vi "XY Graph Cumulative Function of Multiple Plots.vi"(8 "error in (no error)":errorcluster, 10 "Selected Plots":i32[](array[numeric]), 11 "Selected Plot Info":T1) -> (0 "error out":errorcluster, 1 "Cumulative Function Plot Message":string, 3 "Last Cumulative Function Plot":cluster{"t Array":dbl[], "IRF Array":dbl[]}, 4 "Single Plot?":bool)   [LabVIEW 2021, in "XY Graph Add-Ons.lvlib"]
uses:
  XY Graph Add-Ons.lvlib
  XY Graph Selected Plot Info.ctl
  XY Graph Refnum.ctl
  <vilib>/Utility/miscctls.llb/LVPoint32TypeDef.ctl
  Strings/Strings.lvlib
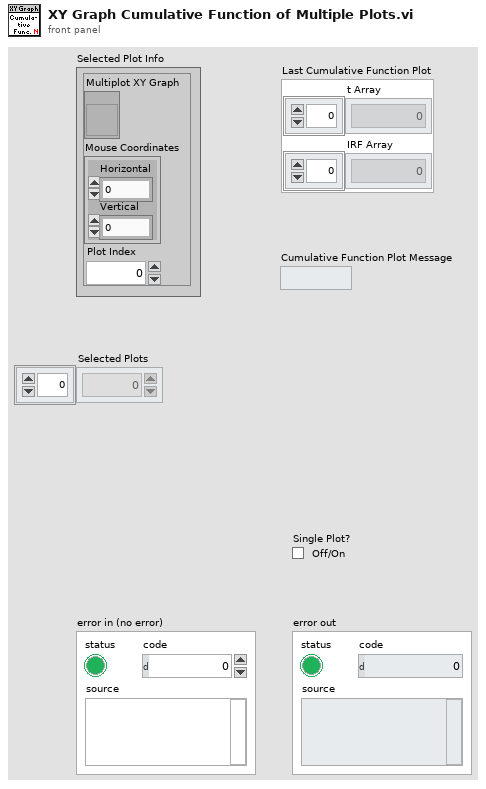
[diagram p1: front panel]
types:
  T1 = typedef "XY Graph Add-Ons.lvlib/XY Graph Selected Plot Info.ctl" = cluster{"Multiplot XY Graph":T2, "Mouse Coordinates":T3, "Plot Index":i32}
  T2 = typedef "XY Graph Add-Ons.lvlib/XY Graph Refnum.ctl" = refnum<vi>
  T3 = typedef "LVPoint32TypeDef.ctl" = cluster{"Horizontal":i32, "Vertical":i32}
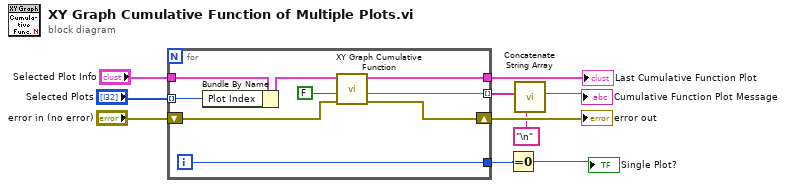
[diagram p0: block diagram]
diagram:
  n1 = for {
    tunnel: "Selected Plot Info" -> [w19]
    tunnel: [w17] -> w5 mode=indexing
    tunnel: [w15] -> w7
    shift-right: [w16] -> w8
    shift-left: "error in (no error)" -> [w18]
    tunnel: "Selected Plots" -> [w13] mode=indexing
    tunnel: [w12] -> w2
    i -> [w12]
    n2 = Bundle By Name(cluster=w19, "Plot Index"=w13) -> (w14:T1)
    n3 = call "XY Graph Cumulative Function.vi"("error in (no error)"=w18, "Replace Plot (T)?"=FALSE, "Selected Plot Info"=w14) -> ("Error Out"=w16:errorcluster, "Cumulative Function Message"=w17:string, "Cumulative Function"=w15:cluster{"t Array":dbl[], "IRF Array":dbl[]})  [unwired: 6 in]
  }
  "error out" <- w8
  "Last Cumulative Function Plot" <- w7
  n4 = Equal To 0?(x=w2) -> (x = 0?=→"Single Plot?":bool)
  n5 = call "Concatenate String Array.vi"("Separator (TAB)"="\n", "String Array"=w5) -> ("Formatted String"=→"Cumulative Function Plot Message":string)  [unwired: 9 in]
